vi "Unsubscribe.vi"(6 "Subscriber Name":string, 7 "Topic Name":string, 8 "error in (no error)":errorcluster, 11 "Message Broker Interface in":refnum<class "Message Broker Interface.lvclass">) -> (0 "error out":errorcluster, 3 "Message Broker Interface out":refnum<class "Message Broker Interface.lvclass">)   [LabVIEW 2016, in "Stream Mediator.lvlib" / "Message Broker Interface.lvclass"]
doc: "--\nCopyright © 2017 Composed SystemsI All rights reserved.\n\nAuthor: Jon McBee <jon.mcbee@composed.io>\n\nThis library is provided \"AS IS\" ,WITHOUT WARRANTIES OR\nCONDITIONS OF ANY KIND, either express or implied.\n\nComposed Systems -- composed.io\n\nStream 0.0.1.1\nJon McBee - Composed Systems\nCopyright (c) 2017, Composed Systems"
uses:
  <userlib>/Composed Systems/Stream/Mediator/Classes/Message Broker Interface/Message Broker Interface.lvclass
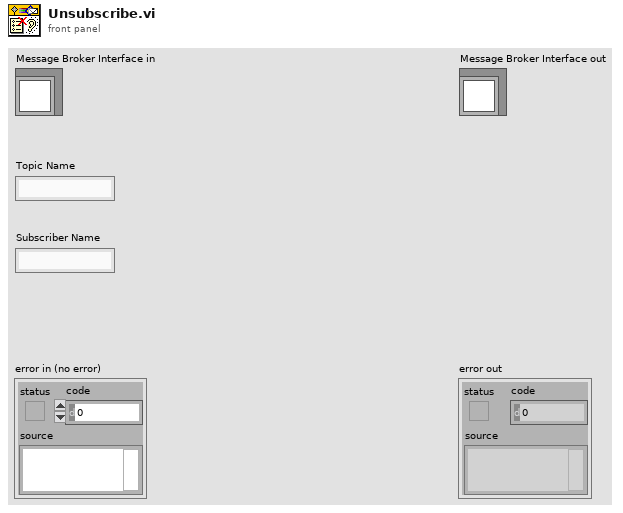
[diagram p1: front panel]
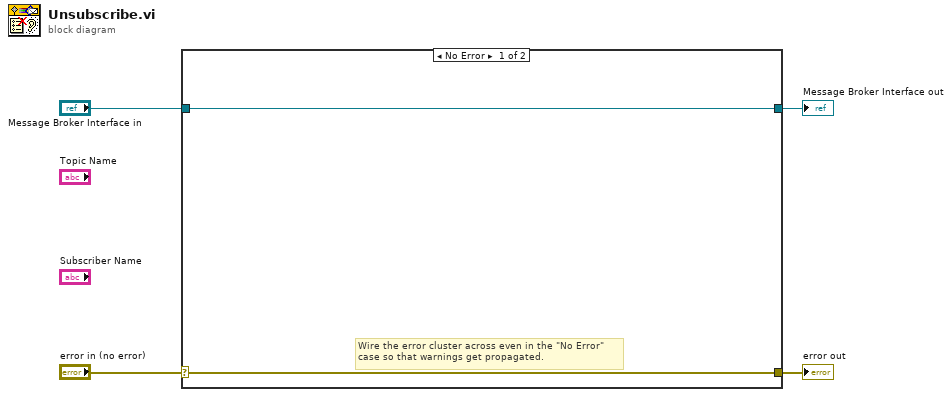
[diagram p0: block diagram]
diagram:
  n1 = case shown="No Error" "error in (no error)" {
    selector: "error in (no error)" -> [w5 w8]
    tunnel: [w5 w8] -> w3
    tunnel: [w6 w7] -> w1
    tunnel: "Message Broker Interface in" -> [w6 w7]
    frame No Error {
      # "Wire the error cluster across even in the \"No Error\"\ncase so that warnings get propagated."
    }
    frame Error {
    }
  }
  "error out" <- w3
  "Message Broker Interface out" <- w1
